vi "Test_Activation.vi"() -> ()   [LabVIEW 2016]
panel:
  out "Activation Function":dbl[][](graph)
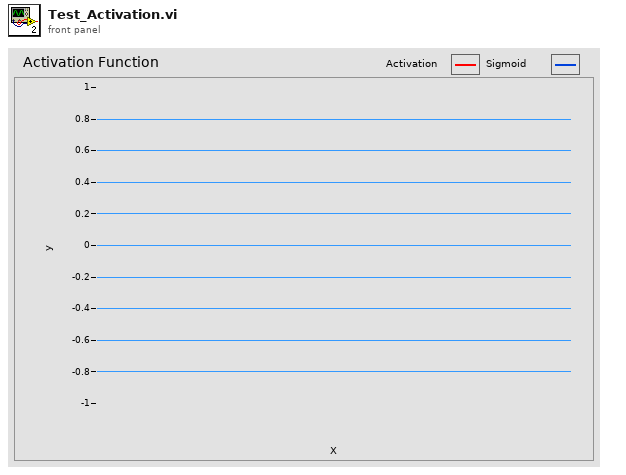
[diagram p1: front panel]
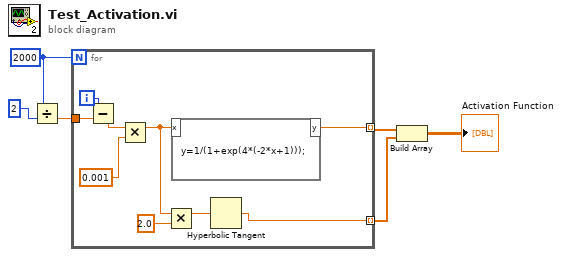
[diagram p0: block diagram]
diagram:
  w3 = 2000
  n1 = Divide(x=w3, y=2 ("x")) -> (x/y=w2:dbl)
  n2 = for {
    N: w3 -> [_]
    tunnel: [w13] -> w6 mode=indexing
    tunnel: [w11] -> w5 mode=indexing
    tunnel: w2 -> [w9]
    i -> [w15]
    n3 = Subtract(x=w15, y=w9) -> (x-y=w10:dbl)
    n4 = Multiply(x=w10, y=0.001) -> (x*y=w12:dbl)
    n5 = Multiply(x=w12, y=2.0) -> (x*y=w8:dbl)
    n6 = formula code="y=1/(1+exp(4*(-2*x+1)));"("x"=w12) -> ("y"=w13:dbl)
    n7 = Hyperbolic Tangent(1:w8) -> (0:w11:dbl)
  }
  n8 = Build Array(w6, w5) -> (→"Activation Function":dbl[][])
